vi "Update Gain Setting.vi"(8 "error in (no error)":errorcluster, 10 "Value":string, 11 "Bobcat 640 in":refnum<class "Bobcat 640.lvclass">) -> (0 "error out":errorcluster, 3 "Bobcat 640 out":refnum<class "Bobcat 640.lvclass">)   [LabVIEW 2018, in "Bobcat 640.lvlib" / "Bobcat 640.lvclass"]
uses:
  Bobcat 640.lvclass
  Bobcat 640.lvclass/Bobcat 640.ctl
  <resource>/objmgr/imaqdx.rc
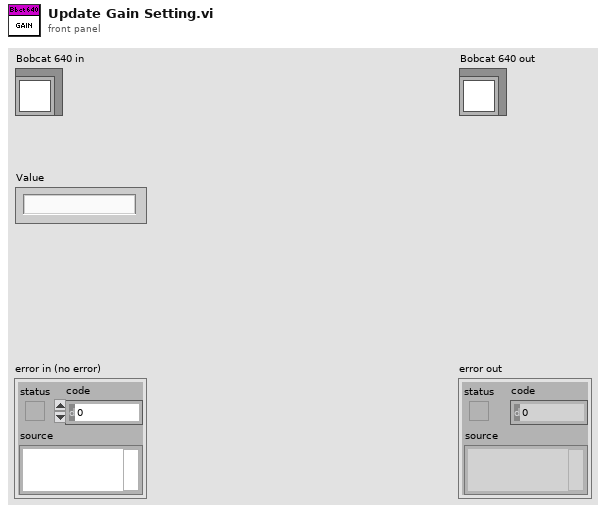
[diagram p1: front panel]
types:
  T1 = typedef "IMAQdx.ctl" = refnum<k21>
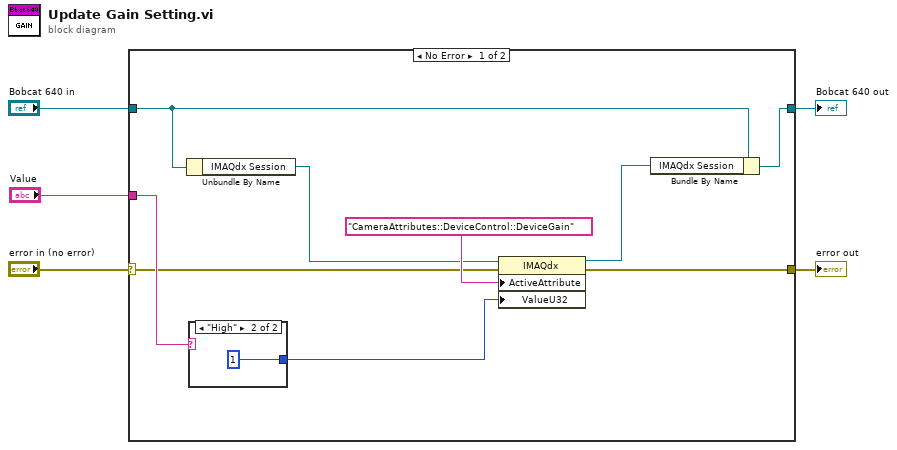
[diagram p0: block diagram]
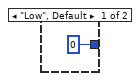
[diagram p2: hidden frame]
diagram:
  n1 = case shown="No Error" "error in (no error)" {
    selector: "error in (no error)" -> [w6 w18]
    tunnel: [w8 w18] -> w4
    tunnel: [w11 w17] -> w2
    tunnel: "Bobcat 640 in" -> [w13 w17]
    tunnel: "Value" -> [w10 _]
    frame No Error {
      n2 = Unbundle By Name(w13) -> ("IMAQdx Session"=w7:T1)
      n3 = case shown="\"High\"" w10 {
        tunnel: [u32 0 ("ValueU32") u32 1 ("ValueU32")] -> w9
        frame "Low", Default {
        }
        frame "High" {
        }
      }
      n4 = property class="IMAQdx"(reference=w7, error in=w6, "ActiveAttribute"="CameraAttributes::DeviceControl::DeviceGain", "ValueU32"=w9) -> (reference out=w12:T1, error out=w8:errorcluster)
      n5 = Bundle By Name(cluster=w13, "IMAQdx Session"=w12) -> (w11:refnum<class "Bobcat 640.lvclass">)
    }
    frame Error {
    }
  }
  "error out" <- w4
  "Bobcat 640 out" <- w2
